vi "DC Voltmeter (Express).vi"() -> ()   [LabVIEW 2015]
panel:
  out "error out":errorcluster
  out "Voltage":dbl
  in  "STOP":bool
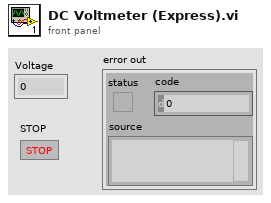
[diagram p1: front panel]
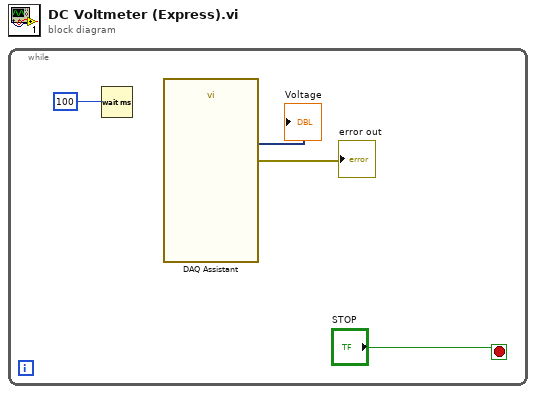
[diagram p0: block diagram]
diagram:
  n1 = while {
    stop <- "STOP" stop-if-true
    n2 = Wait (ms)(milliseconds to wait=u32 100) -> ()  [unwired: 1 out]
    n3 = call "DAQ Assistant"() -> ("data"=→"Voltage":dynamicdata, "error out"=→"error out":errorcluster)  [unwired: 17 in, 1 out]
  }
